vi "Lift Wrapper.vi"(0 "Time":i32=10000, 1 "Down":bool, 2 "Up":bool, 3 "Iterations":i32=1) -> ()   [LabVIEW 2014]
uses:
  Precreated VIs/Robot Global Data.vi
panel:
  in  "Speed":dbl=0.75 format="%#_13g"
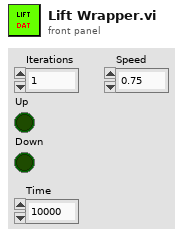
[diagram p1: front panel]
types:
  T1 = cluster{"Limit Switches":cluster{"Lift":cluster{"Top":bool, "High":bool, "Mid":bool, "Low":bool, "Bot":bool}, "Clamp":cluster{"Widest":bool, "Shortest":bool}}, "Ultrasonic":dbl, "Beam Breaker Clamp":bool, "Lift Encoder":dbl}
  T2 = cluster{"Manual Lift":dbl, "Manual Clamp":dbl, "Auto Lift Up":bool, "Auto Lift Down":bool, "Auto Clamp In":bool, "Auto Clamp Out":bool, "Clamp Latch":bool, "Camera LED":bool, "Lift Stop":bool, "Clamp Stop":bool}
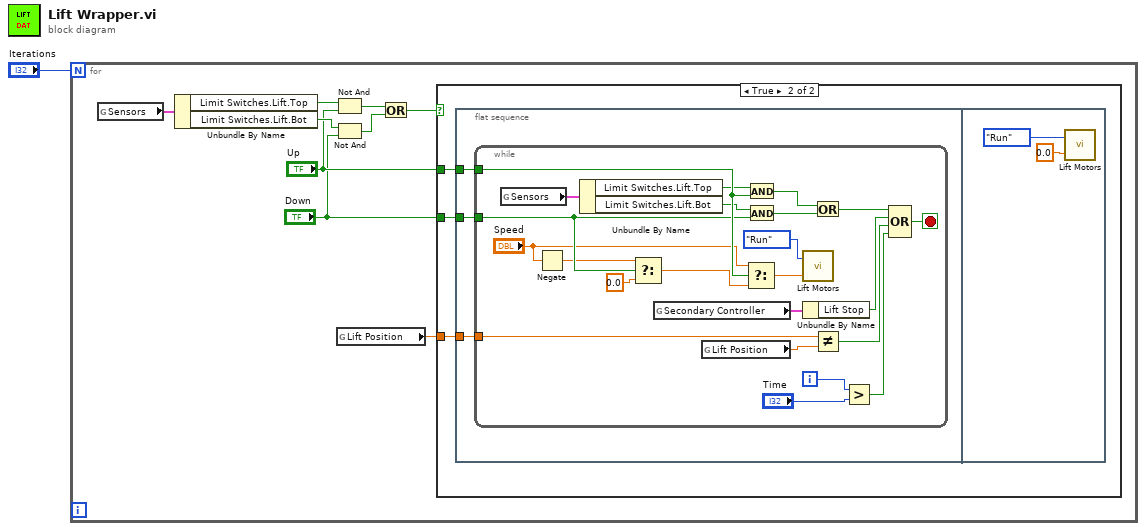
[diagram p0: block diagram]
diagram:
  n1 = for {
    N: "Iterations" -> [_]
    n2 = global read "Robot Global Data.vi" "Sensors"() -> (w6:T1)
    n3 = Unbundle By Name(w6) -> ("Limit Switches.Lift.Top"=w5:bool, "Limit Switches.Lift.Bot"=w4:bool)
    n4 = Not And(1:"Up", 2:w5) -> (0:w10:bool)
    n5 = Not And(1:"Down", 2:w4) -> (0:w9:bool)
    n6 = global read "Robot Global Data.vi" "Lift Position"() -> (w7:dbl)
    n7 = Or(x=w10, y=w9) -> (x .or. y?=w8:bool)
    n8 = case shown="True" w8 {
      tunnel: "Down" -> [_ w13]
      tunnel: "Up" -> [_ w12]
      tunnel: w7 -> [_ w11]
      frame False {
      }
      frame True {
        n9 = flat-sequence {
          tunnel: w13 -> [w16]
          tunnel: w12 -> [w15]
          tunnel: w11 -> [w14]
          frame #0 {
            n10 = while {
              tunnel: w16 -> [w23]
              tunnel: w15 -> [w25]
              tunnel: w14 -> [w36]
              i -> [w30]
              stop <- w27 stop-if-true
              n11 = global read "Robot Global Data.vi" "Sensors"() -> (w26:T1)
              n12 = Negate(x="Speed") -> (-x=w17:dbl)
              n13 = Unbundle By Name(w26) -> ("Limit Switches.Lift.Top"=w24:bool, "Limit Switches.Lift.Bot"=w22:bool)
              n14 = Select(t=w17, s=w23, f=0.0) -> (s? t:f=w38:dbl)
              n15 = global read "Robot Global Data.vi" "Secondary Controller"() -> (w33:T2)
              n16 = global read "Robot Global Data.vi" "Lift Position"() -> (w37:dbl)
              n17 = Select(t="Speed", s=w25, f=w38) -> (s? t:f=w34:dbl)
              n18 = And(x=w24, y=w25) -> (x .and. y?=w20:bool)
              n19 = And(x=w22, y=w23) -> (x .and. y?=w21:bool)
              n20 = call "Lift Motors.vi"("Speed"=w34, "Mode"=enum8{"Start", "Run", "Finish"}."Run") -> ()  [unwired: 1 in]
              n21 = Unbundle By Name(w33) -> ("Lift Stop"=w32:bool)
              n22 = Or(x=w20, y=w21) -> (x .or. y?=w19:bool)
              n23 = Not Equal?(x=w36, y=w37) -> (x != y?=w31:bool)
              n24 = Greater?(x=w30, y="Time") -> (0:w28:bool)
              n25 = Compound Arithmetic op=OR(w19, w32, w31, w28) -> (w27:bool)
            }
          }
          frame #1 {
            n26 = call "Lift Motors.vi"("Speed"=0.0, "Mode"=enum8{"Start", "Run", "Finish"}."Run") -> ()  [unwired: 1 in]
          }
        }
      }
    }
  }
